vi "Apply.vi"(8 "error in":errorcluster, 11 "Thermometer DAQmx RTD Cont CFG in":refnum<class "Thermometer DAQmx RTD Cont CFG Simulated.lvclass">) -> (0 "error out":errorcluster, 3 "Thermometer DAQmx RTD Cont CFG out":refnum<class "Thermometer DAQmx RTD Cont CFG Simulated.lvclass">)   [LabVIEW 2024, in "DAQmx Simulated CFGs.lvlib" / "Thermometer DAQmx RTD Cont CFG Simulated.lvclass"]
uses:
  Thermometer DAQmx RTD Cont CFG Simulated.lvclass
  Configurations/CFG Base/CFG Base.lvclass/CFG Base.ctl
  Thermometer DAQmx RTD Cont CFG/Thermometer DAQmx RTD Cont CFG.lvclass
  Configurations/CFG Base/CFG Base.lvclass
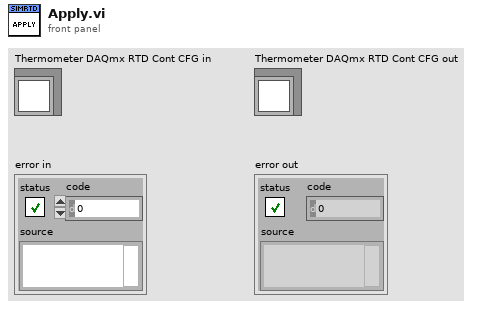
[diagram p1: front panel]
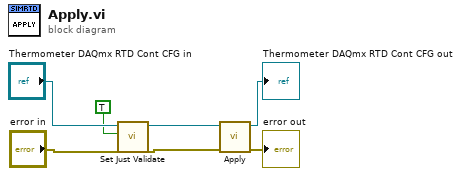
[diagram p0: block diagram]
diagram:
  n1 = call "Set Just Validate.vi"("Just Validate"=TRUE, "CFG Base in"="Thermometer DAQmx RTD Cont CFG in") -> ("CFG Base out"=w3:refnum<class "Thermometer DAQmx RTD Cont CFG Simulated.lvclass">)  [unwired: 9 in]
  n2 = call-parent "Apply.vi"("error in"="error in", "Thermometer DAQmx RTD Cont CFG in"=w3) -> ("error out"=→"error out":errorcluster, "Thermometer DAQmx RTD Cont CFG out"=→"Thermometer DAQmx RTD Cont CFG out":refnum<class "Thermometer DAQmx RTD Cont CFG Simulated.lvclass">)  [unwired: 8 in]
